vi "Untitled 9 (SubVI).vi"(9 "Кол-во копий":i32, 10 "Размер окна с паузами":i32, 11 "см. 1.5 in":dbl[][](array[numeric])) -> (3 "см. 1.5 out":dbl[](array[numeric]))   [LabVIEW 2017]
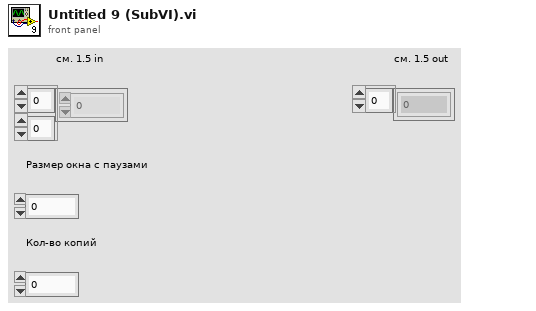
[diagram p1: front panel]
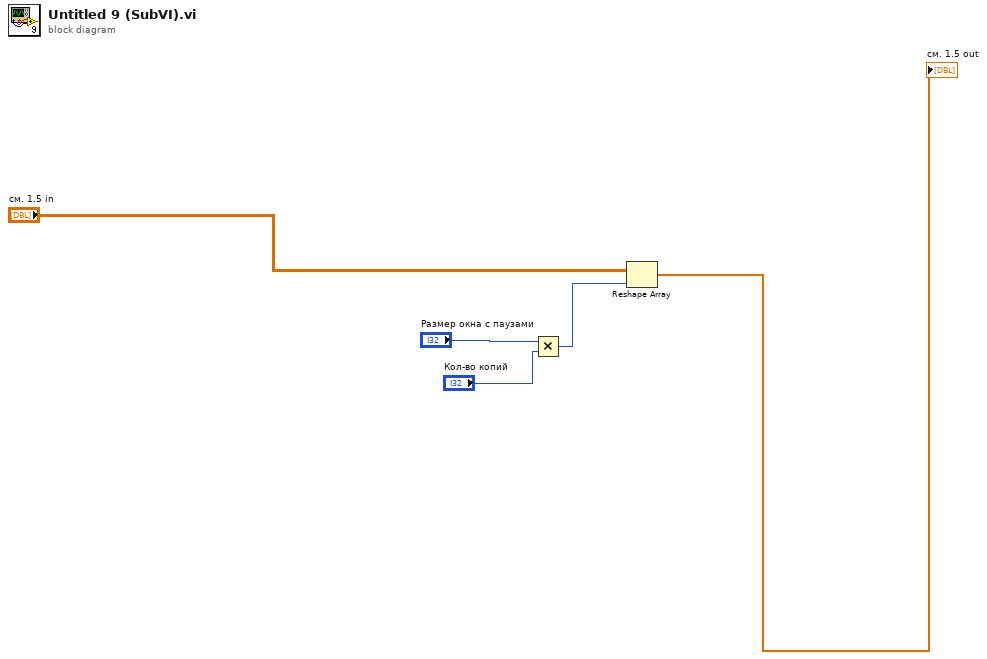
[diagram p0: block diagram]
diagram:
  n1 = Multiply(x="Размер окна с паузами", y="Кол-во копий") -> (x*y=w3:i32)
  n2 = Reshape Array("см. 1.5 in", w3) -> (→"см. 1.5 out":dbl[])
